vi "Read Gannt Chart.vi"(8 "error in (no error)":errorcluster, 11 "GanntChart in":refnum<class "GanntChart.lvclass">) -> (0 "error out":errorcluster, 2 "Gannt Chart":T1[][](array[typedef]), 3 "GanntChart out":refnum<class "GanntChart.lvclass">)   [LabVIEW 2013, in "GanntChart.lvclass"]
uses:
  GanntChart.lvclass
  Controls/GanntChart_Element.ctl
  GanntChart.lvclass/GanntChart.ctl
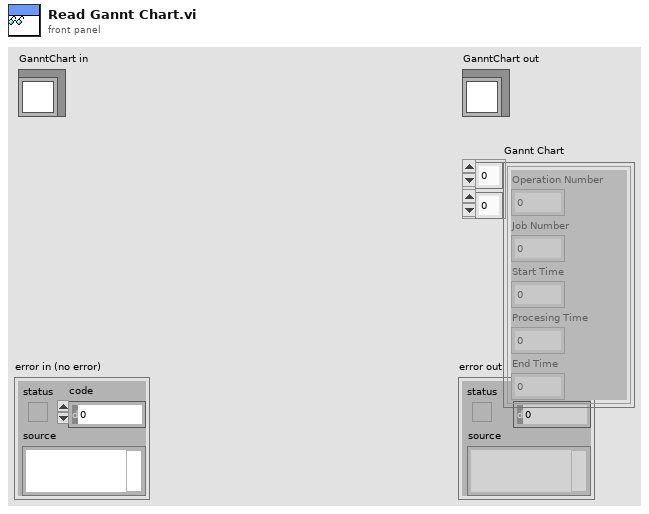
[diagram p1: front panel]
types:
  T1 = typedef "GanntChart_Element.ctl" = cluster{"Operation Number":i32, "Job Number":i32, "Start Time":i32, "Procesing Time":u16, "End Time":i32}
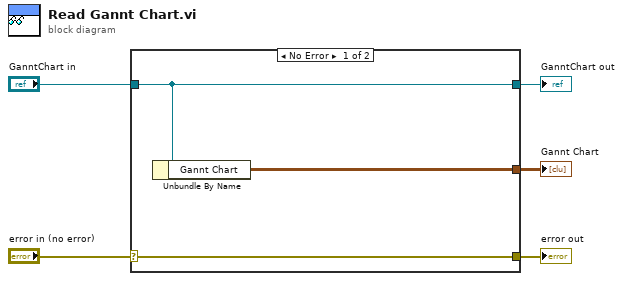
[diagram p0: block diagram]
diagram:
  n1 = case shown="No Error" "error in (no error)" {
    selector: "error in (no error)" -> [w8 w9]
    tunnel: [w8 w9] -> w4
    tunnel: [w7 w10] -> w2
    tunnel: "GanntChart in" -> [w7 w10]
    tunnel: [w6 _] -> w1
    frame No Error {
      n2 = Unbundle By Name(w7) -> ("Gannt Chart"=w6:T1[][])
    }
    frame Error {
    }
  }
  "error out" <- w4
  "GanntChart out" <- w2
  "Gannt Chart" <- w1
